vi "game_screen.vi"() -> ()   [LabVIEW 2025]
panel:
  in  "stop":bool
  out "Boolean 4":bool
  out "Boolean 3":bool
  out "Boolean 2":bool
  out "Boolean":bool
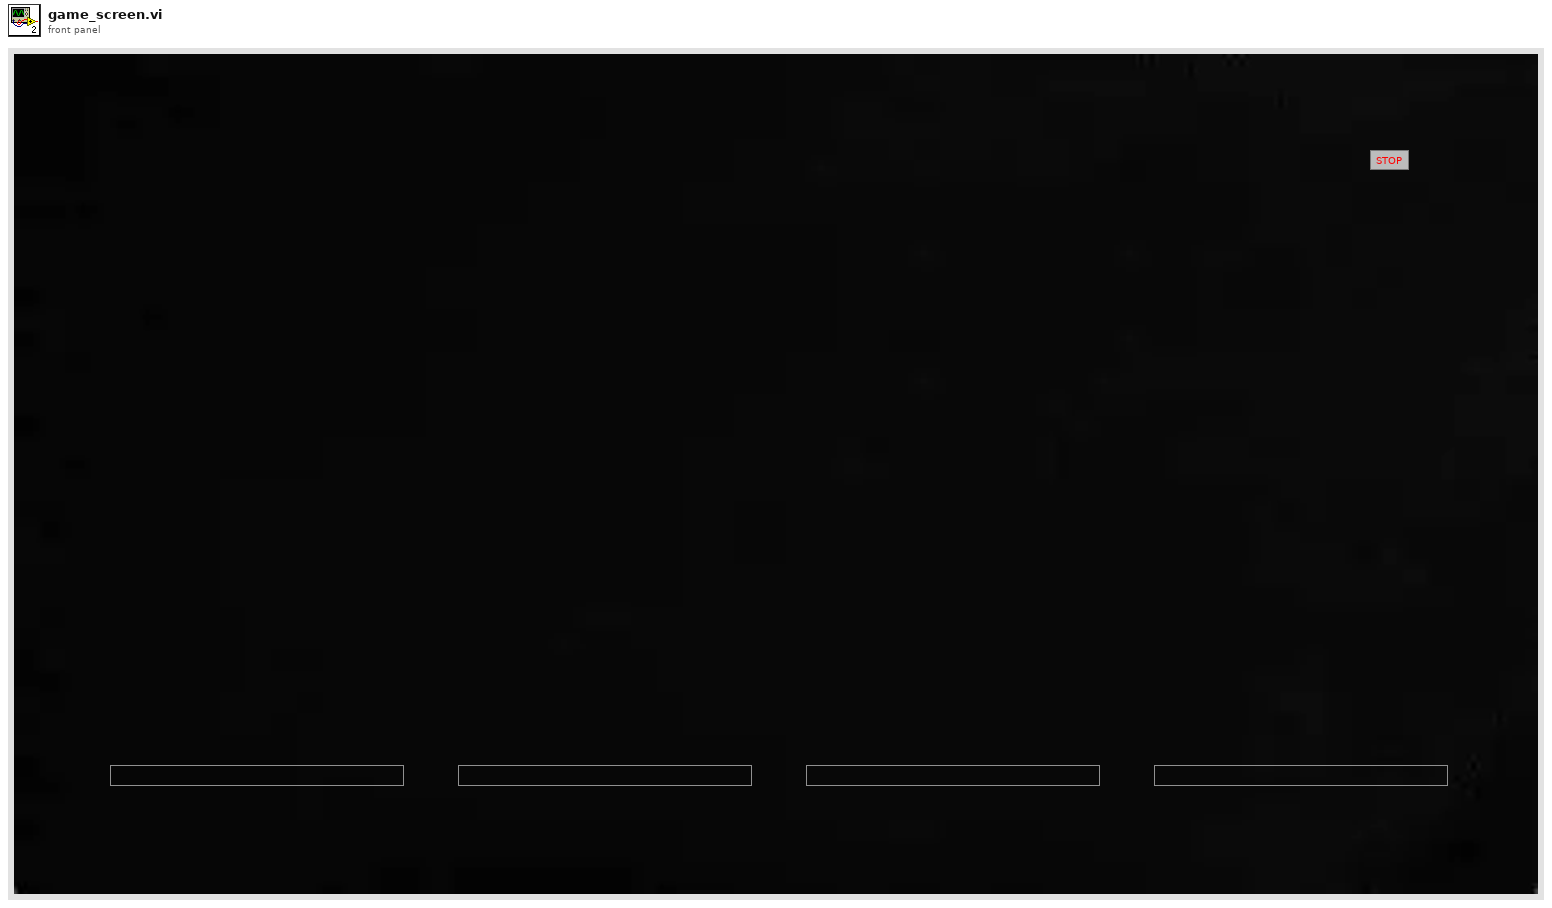
[diagram p1: front panel]
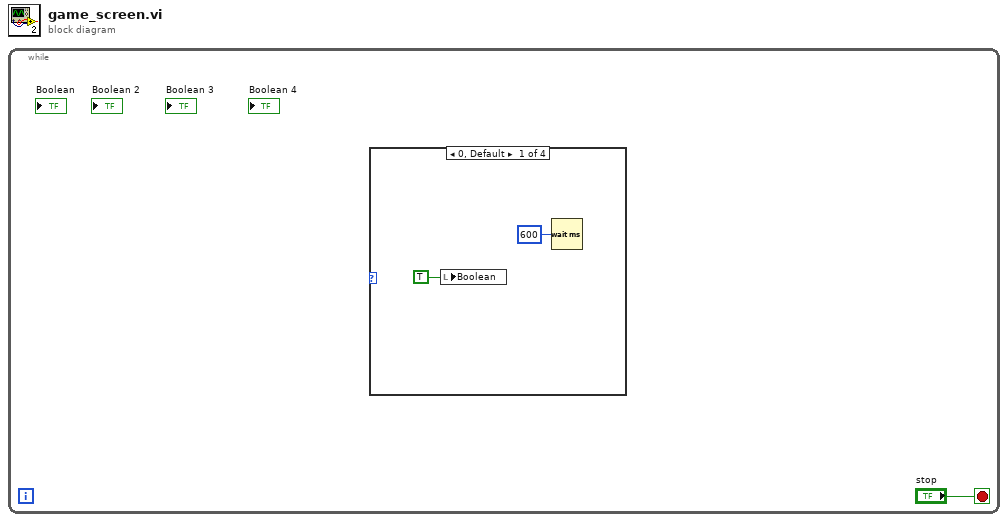
[diagram p0: block diagram]
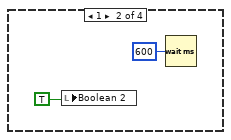
[diagram p2: hidden frame]
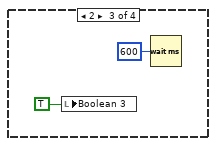
[diagram p3: hidden frame]
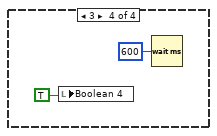
[diagram p4: hidden frame]
diagram:
  n1 = while {
    stop <- "stop" stop-if-true
    n2 = case shown="0, Default" {
      selector: _ -> [_ _ _ _]
      frame 0, Default {
        n3 = local write "Boolean"(TRUE) -> ()
        n4 = Wait (ms)(milliseconds to wait=u32 600) -> ()  [unwired: 1 out]
      }
      frame 1 {
        n5 = local write "Boolean 2"(TRUE) -> ()
        n6 = Wait (ms)(milliseconds to wait=u32 600) -> ()  [unwired: 1 out]
      }
      frame 2 {
        n7 = local write "Boolean 3"(TRUE) -> ()
        n8 = Wait (ms)(milliseconds to wait=u32 600) -> ()  [unwired: 1 out]
      }
      frame 3 {
        n9 = local write "Boolean 4"(TRUE) -> ()
        n10 = Wait (ms)(milliseconds to wait=u32 600) -> ()  [unwired: 1 out]
      }
    }
  }
